vi "Launch One-Button Dialog Box.vi"(6 "Modal? (T)":bool=TRUE, 7 "Return Message (Optional)":refnum<class "Dialog Return Msg.lvclass">, 9 "Button Text (OK)":string="OK", 10 "Message Text":string, 11 "Dialog Launcher":refnum<class "IViewable.lvclass">) -> (0 "error out":errorcluster)   [LabVIEW 2017, in "OneButtonDialogBox.lvlib" / "OneButtonDialogBox.lvclass"]
doc: "<License>\nCopyright © 2017 Composed Systems, LLC | All rights reserved\nwww.composed.io\n\nAuthor: Ethan Stern <ethan.stern@composed.io>\n\nThis software is provided \"AS IS\" WITHOUT WARRANTIES, either express or implied, AND IS FOR EDUCATIONAL PURPOSES ONLY.\n</License>"
uses:
  OneButtonDialogBox.lvclass
  Framework/IViewable/IViewable/IViewable.lvclass
  C:/Program Files (x86)/National Instruments/LabVIEW 2017/vi.lib/ActorFramework/Actor/Actor.lvclass
  Framework/IDialogBox/IDialogBox Messages/Dialog Return Msg/Dialog Return Msg.lvclass
  C:/Git/mva-framework/Source/Framework/IDialogBox/IDialogBox/IDialogBox.lvclass
  OneButtonDialogBox.lvclass/OneButtonDialogBox.ctl
  <vilib>/ActorFramework/Actor/Actor.lvclass/Actor.ctl
  <vilib>/ActorFramework/Message Enqueuer/Message Enqueuer.lvclass/Message Enqueuer.ctl
  Framework/IViewable/IViewable Messages/Launch Dialog Box Msg/Launch Dialog Box Msg.lvclass/Launch Dialog Box Msg.ctl
  <vilib>/ActorFramework/Message Enqueuer/Init from Existing Queue.vi
  <vilib>/ActorFramework/Message Enqueuer/Enqueue.vi
  Framework/IViewable/IViewable Messages/Launch Dialog Box Msg/Launch Dialog Box Msg.lvclass
  C:/Program Files (x86)/National Instruments/LabVIEW 2017/vi.lib/ActorFramework/Message/Message.lvclass
  <vilib>/ActorFramework/Message Priority Queue/Priority Enqueue.vi
  <vilib>/ActorFramework/Message Enqueuer/Message Enqueuer.lvclass
  <vilib>/ActorFramework/Actor/Actor.lvclass
panel:
  in  "error in (no error)":errorcluster
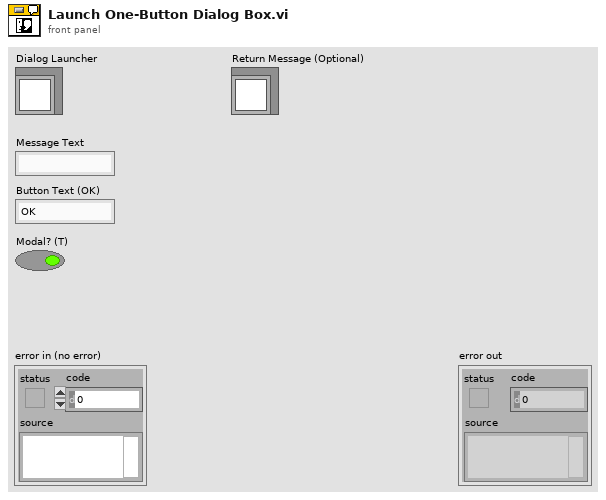
[diagram p1: front panel]
types:
  T1 = enum32{"Invalid", "Default", "Floating", "Floating/Auto-Hide", "Modal"}
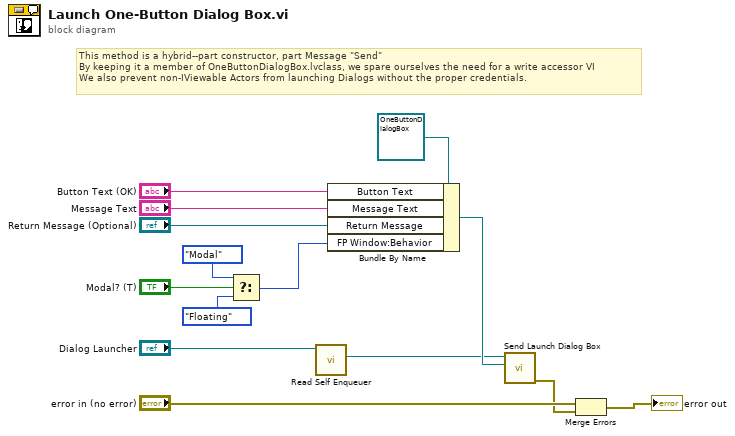
[diagram p0: block diagram]
diagram:
  # "This method is a hybrid--part constructor, part Message \"Send\"\nBy keeping it a member of OneButtonDialogBox.lvclass, we spare ourselves the need for a write accessor VI\nWe also prevent non-IViewable Actors from launching Dialogs without the proper credentials."
  n1 = Select(t=T1."Modal" ("FP Window:Behavior"), s="Modal? (T)", f=T1."Floating" ("FP Window:Behavior")) -> (s? t:f=w3:T1)
  n2 = call <vilib>:"Read Self Enqueuer.vi"("Actor"="Dialog Launcher") -> ("Self Enqueuer"=w5:refnum<class "Message Enqueuer.lvclass">)  [unwired: 10 in]
  n3 = Bundle By Name(cluster=refnum<class "OneButtonDialogBox.lvclass"> refnum ("OneButtonDialogBox in"), "Button Text"="Button Text (OK)", "Message Text"="Message Text", "Return Message"="Return Message (Optional)", "FP Window:Behavior"=w3) -> (w9:refnum<class "OneButtonDialogBox.lvclass">)
  n4 = call "Send Launch Dialog Box.vi"("DialogBox"=w9, "Message Enqueuer"=w5) -> ("error out"=w10:errorcluster)  [unwired: 8 in, 1 out]
  n5 = Merge Errors("error in (no error)", w10) -> (→"error out":errorcluster)
